vi "PSCreateSnippet.vi"(8 "error in (no error)":errorcluster, 10 "PNG Path":path, 11 "VI Path":path) -> (0 "error out":errorcluster, 2 "PNG Path out":path, 3 "VI Path out":path)   [LabVIEW 2013, in "VIVendor.lvlib" / "VVPngSnippet.lvlib"]
doc: "Embeds the block diagram from a VI into a PNG file.\n\nOrigin:\n* PNG Snippet VIs from Code Complete Tool\n* http://sourceforge.net/projects/lv-cct-tool/\n* Commit: 9d97aea5cbd2fc456c5914801e927df6a901d523\n* License: BSD -- see NOTICE.txt"
uses:
  VVPngSnippet.lvlib
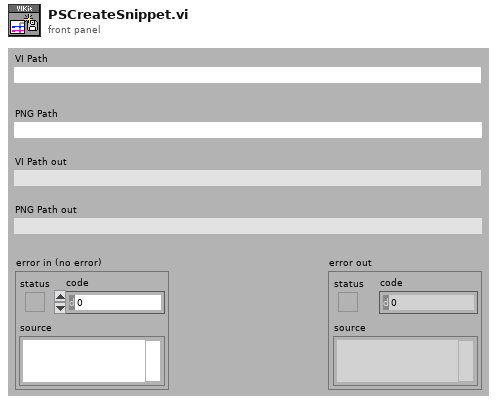
[diagram p1: front panel]
types:
  T1 = enum16{"open", "replace", "create", "open or create", "replace or create", "replace or create with confirmation"}
  T2 = cluster{"Year":u16, "Month":u8, "Day":u8, "Hour":u8, "Minute":u8, "Second":u8}
  T3 = enum16{"open", "open or create", "create or replace", "create", "open (read only)"}
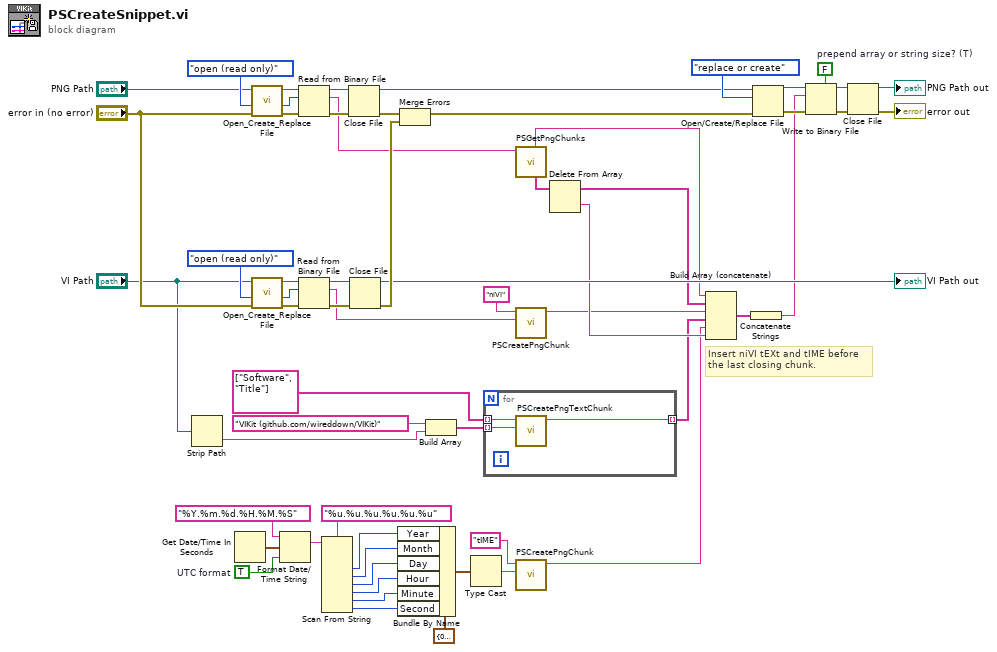
[diagram p0: block diagram]
diagram:
  w19 = TRUE  # UTC format
  w20 = FALSE  # prepend array or string size? (T)
  # "Insert niVI tEXt and tIME before the last closing chunk."
  n1 = Strip Path(path="VI Path") -> (name=w18:string)  [unwired: 1 out]
  n2 = Get Date/Time In Seconds() -> (seconds since 1Jan1904=w38:timestamp)
  n3 = call <vilib>:"Open_Create_Replace File.vi"("error in (no error)"="error in (no error)", "function (open:0)"=T3."open (read only)", "file path"="PNG Path") -> ("error out"=w47:errorcluster, "file size (bytes)"=w22:i32, "refnum"=w46:refnum<file>)  [unwired: 5 in, 1 out]
  n4 = call <vilib>:"Open_Create_Replace File.vi"("error in (no error)"="error in (no error)", "function (open:0)"=T3."open (read only)", "file path"="VI Path") -> ("error out"=w44:errorcluster, "file size (bytes)"=w42:i32, "refnum"=w43:refnum<file>)  [unwired: 5 in, 1 out]
  n5 = Format Date/Time String(time format string (%c)="%Y.%m.%d.%H.%M.%S", seconds (now)=w38, UTC format=w19) -> (date/time string=w36:string)
  n6 = Read from Binary File(8:w47, 10:w22, 11:w46) -> (0:w49:errorcluster, 2:w10:string, 3:w50:refnum<file>)  [unwired: 3 in, 1 out]
  n7 = Read from Binary File(8:w44, 10:w42, 11:w43) -> (0:w58:errorcluster, 2:w56:string, 3:w59:refnum<file>)  [unwired: 3 in, 1 out]
  n8 = Scan From String(format string="%u.%u.%u.%u.%u.%u", input string=w36) -> (output 1=w34:u32, output 2=w33:u32, output 3=w32:u32, output 4=w31:u32, output 5=w30:u32, output 6=w29:u32)  [unwired: 8 in, 3 out]
  n9 = Close File(refnum=w50, error in=w49) -> (path=w11:path, error out=w13:errorcluster)
  n10 = Close File(refnum=w59, error in=w58) -> (path=→"VI Path out":path, error out=w12:errorcluster)
  n11 = Bundle By Name(cluster=T2 {"Year"=0, "Month"=0, "Day"=0, "Hour"=0, "Minute"=0, "Second"=0}, "Year"=w34, "Month"=w33, "Day"=w32, "Hour"=w31, "Minute"=w30, "Second"=w29) -> (w39:T2)
  n12 = Merge Errors(w13, w12) -> (w24:errorcluster)
  n13 = Build Array("VIKit (github.com/wireddown/VIKit)", w18) -> (w26:string[])
  n14 = Type Cast(x=w39) -> (*(type *) &x=w40:string)  [unwired: 1 in]
  n15 = for {
    tunnel: [w62] -> w2 mode=indexing
    tunnel: w26 -> [w61] mode=indexing
    tunnel: string[] ["Software", "Title"] -> [w60] mode=indexing
    n16 = call "PSCreatePngTextChunk.vi"("Contents"=w61, "Keyword"=w60) -> ("PNG Chunk"=w62:string)  [unwired: 9 in]
  }
  n17 = call "PSGetPngChunks.vi"("data"=w10) -> ("Chunks"=w55:string[], "Header"=w5:string)  [unwired: 5 in, 4 out]
  n18 = call "PSCreatePngChunk.vi"("Data"=w56, "Name"="niVI" ("element")) -> ("PNG Chunk"=w1:string)  [unwired: 9 in]
  n19 = call "PSCreatePngChunk.vi"("Data"=w40, "Name"="tIME") -> ("PNG Chunk"=w3:string)  [unwired: 9 in]
  n20 = Delete From Array(array=w55) -> (deleted portion=w7:string, array with subset deleted=w6:string[])  [unwired: 2 in]
  n21 = Build Array (concatenate)(w5, w6, w1, w2, w3, w7) -> (w52:string[])
  n22 = Concatenate Strings(w52) -> (w4:string)
  n23 = Open/Create/Replace File(file path (use dialog)=w11, error in=w24, operation (0:open)=T1."replace or create") -> (refnum out=w25:refnum<file>, error out=w23:errorcluster)  [unwired: 3 in, 1 out]
  n24 = Write to Binary File ("Write File")(file (use dialog)=w25, data=w4, error in=w23, 5:w20) -> (refnum out=w53:refnum<file>, error out=w54:errorcluster)  [unwired: 2 in, 1 out]
  n25 = Close File(refnum=w53, error in=w54) -> (path=→"PNG Path out":path, error out=→"error out":errorcluster)
